vi "picoscopeInitializeAcquisition.vi"(6 "nSegmentsInt":i32, 7 "nSegments":T1 format="%.4p", 8 "error in (no error)":errorcluster, 9 "Use Serial Number":bool, 10 "Serial Number":string, 11 "PicoscopeV2 in":refnum<class "PicoscopeV2.lvclass">) -> (0 "error out":errorcluster, 1 "Device Info":T2, 2 "USB Powered":bool, 3 "PicoscopeV2 out":refnum<class "PicoscopeV2.lvclass">, 4 "enabled array":i16[](array[numeric]), 5 "USB 3.0 device on non-USB 3.0 Port":bool)   [LabVIEW 2020, in "PicoscopeV2.lvclass"]
uses:
  PicoscopeV2.lvclass
  nSegments.ctl
  PicoscopeV2.lvclass/PicoscopeV2.ctl
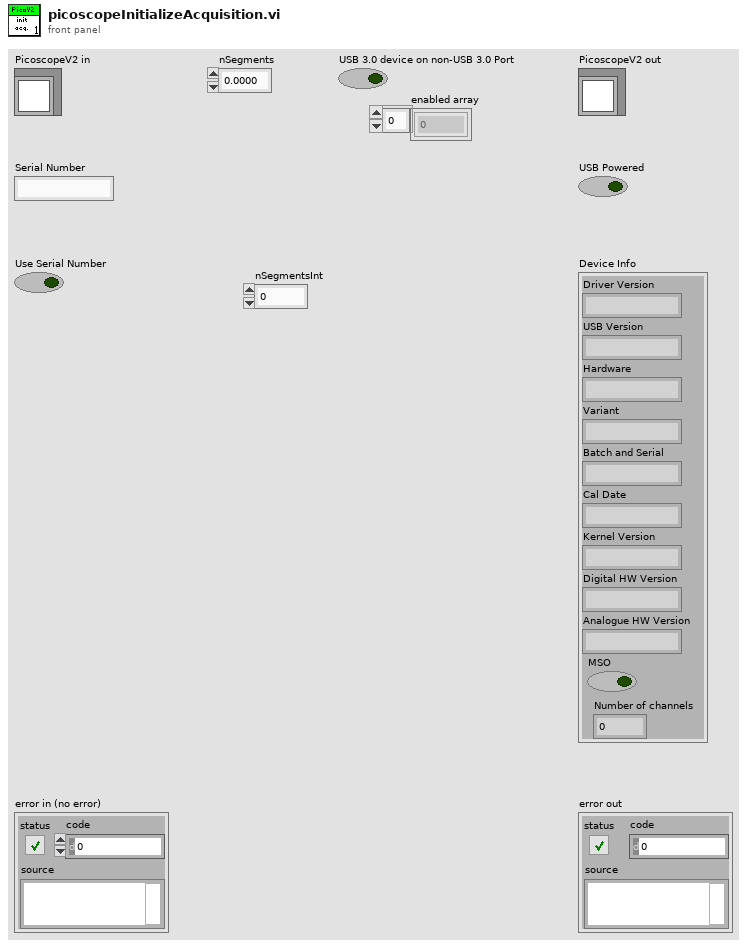
[diagram p1: front panel]
types:
  T1 = typedef "nSegments.ctl" = u64
  T2 = cluster{"Driver Version":string, "USB Version":string, "Hardware":string, "Variant":string, "Batch and Serial":string, "Cal Date":string, "Kernel Version":string, "Digital HW Version":string, "Analogue HW Version":string, "MSO":bool, "Number of channels":i16}
  T3 = cluster{"Trigger Enabled":bool, "Trigger Source":enum16{"Channel A", "Channel B", "Channel C", "Channel D", "Ext."}, "Trigger Threshold (volts)":dbl, "Trigger Direction":u16, "Trigger Delay (samples)":u32, "Auto Trigger Time (ms)":i16}
  T4 = typedef "PicoScope5000aDigitalChannelSettings.ctl" = cluster{"Enabled":bool, "Logic Level":i16}
  T5 = typedef "PicoScope5000aAnalogChannelSettings.ctl" = cluster{"Enabled":bool, "Coupling":i16, "Range":u16, "Analogue Offset":sgl, "Bandwidth Limit":u32}
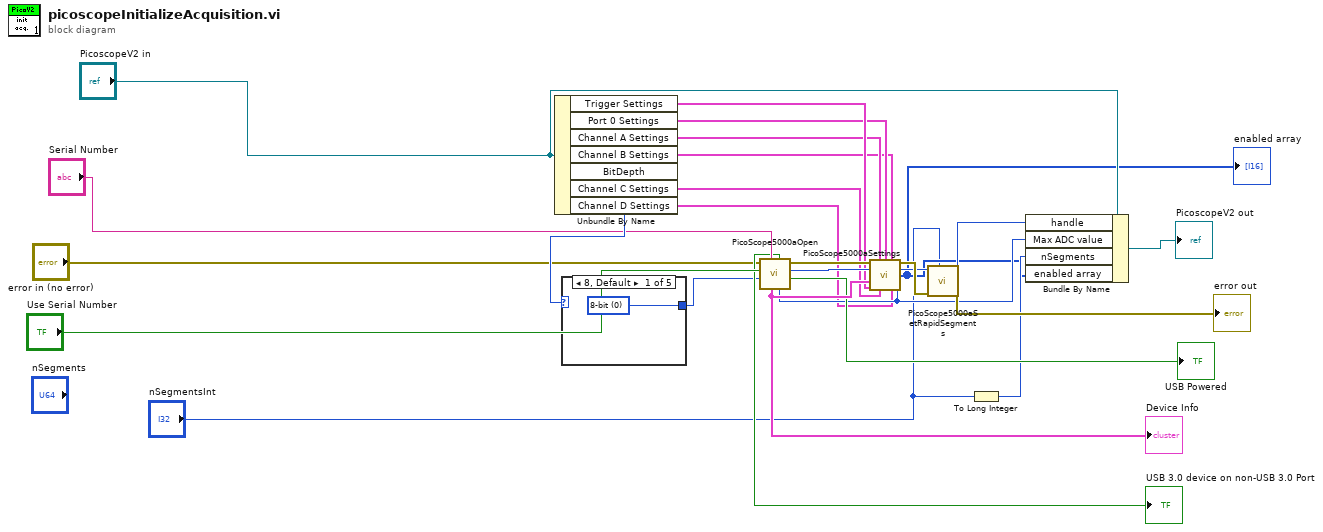
[diagram p0: block diagram]
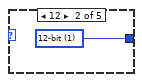
[diagram p2: hidden frame]
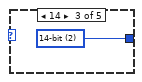
[diagram p3: hidden frame]
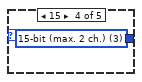
[diagram p4: hidden frame]
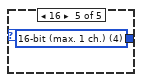
[diagram p5: hidden frame]
diagram:
  n1 = Unbundle By Name("PicoscopeV2 in") -> ("Trigger Settings"=w8:T3, "Port 0 Settings"=w7:T4, "Channel A Settings"=w6:T5, "Channel B Settings"=w4:T5, "BitDepth"=w26:i32, "Channel C Settings"=w2:T5, "Channel D Settings"=w1:T5)
  n2 = case shown="8, Default" w26 {
    tunnel: [w27 w28 w29 w30 w31] -> w9
    frame 8, Default {
      w27 = 0 items=["8-bit", "12-bit", "14-bit", "15-bit (max. 2 ch.)", "16-bit (max. 1 ch.)"] ("Resolution")
    }
    frame 12 {
      w28 = 1 items=["8-bit", "12-bit", "14-bit", "15-bit (max. 2 ch.)", "16-bit (max. 1 ch.)"] ("Resolution")
    }
    frame 14 {
      w29 = 2 items=["8-bit", "12-bit", "14-bit", "15-bit (max. 2 ch.)", "16-bit (max. 1 ch.)"] ("Resolution")
    }
    frame 15 {
      w30 = 3 items=["8-bit", "12-bit", "14-bit", "15-bit (max. 2 ch.)", "16-bit (max. 1 ch.)"] ("Resolution")
    }
    frame 16 {
      w31 = 4 items=["8-bit", "12-bit", "14-bit", "15-bit (max. 2 ch.)", "16-bit (max. 1 ch.)"] ("Resolution")
    }
  }
  n3 = call "PicoScope5000aOpen.vi"("Serial Number"="Serial Number", "Resolution"=w9, "Use Serial Number"="Use Serial Number", "error in (no error)"="error in (no error)") -> ("USB Powered"=→"USB Powered":bool, "handle"=w18:i16, "error out"=w19:errorcluster, "Max ADC value"=w11:i16, "USB 3.0 device on non-USB 3.0 Port"=→"USB 3.0 device on non-USB 3.0 Port":bool, "Device Info"=w22:T2)  [unwired: 2 in]
  "Device Info" <- w22
  n4 = call "PicoScope5000aSettings.vi"("error in"=w19, "Channel A Settings"=w6, "Port 0 Settings"=w7, "Channel B Settings"=w4, "handle in"=w18, "Device Info"=w22, "Trigger Settings"=w8, "Channel C Settings"=w2, "Channel D Settings"=w1, "Max ADC value"=w11) -> ("error out"=w17:errorcluster, "handle out"=w16:i16, "enabled array"=w5:i16[])  [unwired: 3 in]
  "enabled array" <- w5
  n5 = call "PicoScope5000aSetRapidSegments.vi"("nSegments"="nSegmentsInt", "error in (no error)"=w17, "handle in"=w16) -> ("error out"=→"error out":errorcluster, "handle out"=w12:i16)  [unwired: 6 in, 1 out]
  n6 = To Long Integer(number="nSegmentsInt") -> (32bit integer=w10:i32)
  n7 = Bundle By Name(cluster="PicoscopeV2 in", "handle"=w12, "Max ADC value"=w11, "nSegments"=w10, "enabled array"=w5) -> (→"PicoscopeV2 out":refnum<class "PicoscopeV2.lvclass">)
